vi "MaskPayload.vi"(5 "mask value":u32 format="%.0x", 8 "payload":string) -> (2 "masked payload":string)   [LabVIEW 2014, in "Websocket.lvlib"]
uses:
  Websocket.lvlib
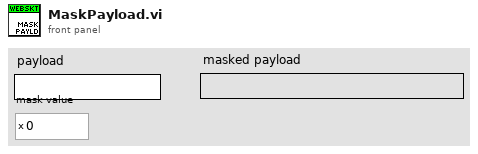
[diagram p1: front panel]
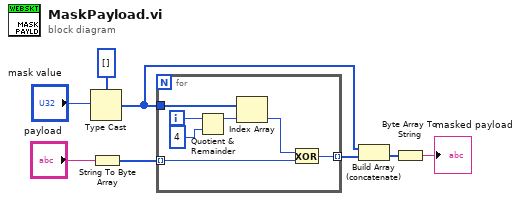
[diagram p0: block diagram]
diagram:
  n1 = Type Cast(type=u8[] [], x="mask value") -> (*(type *) &x=w2:u8[])
  n2 = String To Byte Array(string="payload") -> (unsigned byte array=w5:u8[])
  n3 = for {
    tunnel: w2 -> [w15]
    tunnel: w5 -> [w11] mode=indexing
    tunnel: [w9] -> w3 mode=indexing
    i -> [w13]
    n4 = Quotient & Remainder(x=w13, y=4) -> (x-y*floor(x/y)=w14:i32)  [unwired: 1 out]
    n5 = Index Array(array=w15, index=w14) -> (element=w10:u8)
    n6 = Exclusive Or(1:w11, 2:w10) -> (0:w9:u8)
  }
  n7 = Build Array (concatenate)(w2, w3) -> (w1:u8[])
  n8 = Byte Array To String(unsigned byte array=w1) -> (string=→"masked payload":string)
